vi "Convert ASCII to Unicode.vi"(4 "ASCII String In":string) -> (1 "Unicode String Out":string)   [LabVIEW 2012]
doc: "Convert an ASCII string to Unicode.\n\nChristopher G. Relf\nCertified LabVIEW Architect\nchristopher_relf@yahoo.com\nCopyright (c) 2004 - All Rights Reserved\n\nLicense:\nThis code is owned by Christopher G. Relf and is licensed under the Creative Commons License. See http://creativecommons.org for full license terms.\n\nThis VI is LAVA Certified. For more information, visit http://forums.lavag.org."
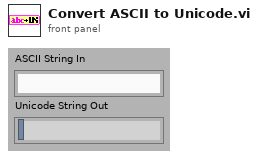
[diagram p1: front panel]
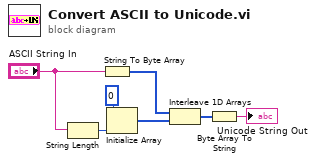
[diagram p0: block diagram]
diagram:
  n1 = String Length(string="ASCII String In") -> (length=w4:i32)
  n2 = String To Byte Array(string="ASCII String In") -> (unsigned byte array=w2:u8[])
  n3 = Initialize Array(u8 0, w4) -> (w1:u8[])
  n4 = Interleave 1D Arrays(w2, w1) -> (w3:u8[])
  n5 = Byte Array To String(unsigned byte array=w3) -> (string=→"Unicode String Out":string)
